vi "Set Btn BG.vi"(8 "error in (no error)":errorcluster, 10 "BG Color":u32(colorbox), 11 "[V] Main UI in":refnum<class "[V] Main UI.lvclass">) -> (0 "error out":errorcluster, 3 "[V] Main UI out":refnum<class "[V] Main UI.lvclass">)   [LabVIEW 2020, in "[V] Main UI.lvlib" / "[V] Main UI.lvclass"]
uses:
  [V] Main UI.lvclass
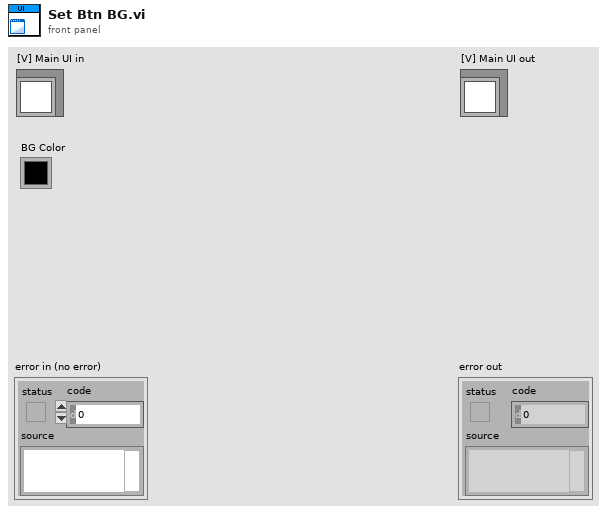
[diagram p1: front panel]
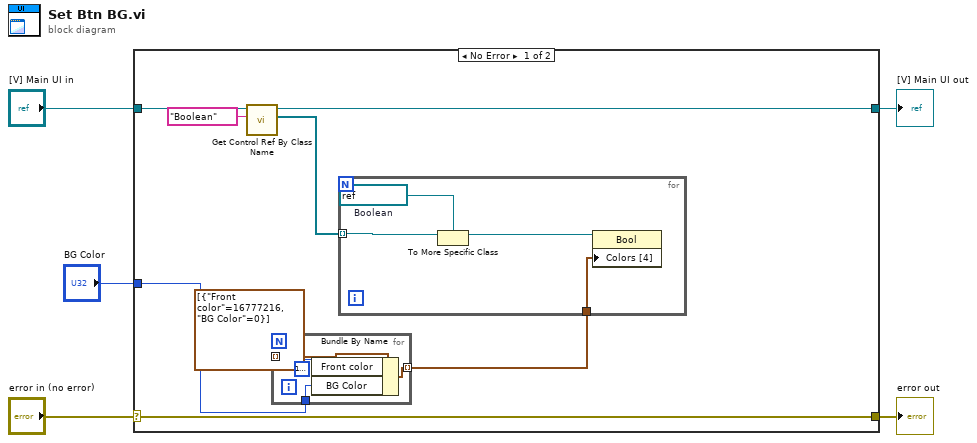
[diagram p0: block diagram]
diagram:
  n1 = case shown="No Error" "error in (no error)" {
    selector: "error in (no error)" -> [w13 w23]
    tunnel: [w13 w23] -> w4
    tunnel: [w10 w22] -> w2
    tunnel: "[V] Main UI in" -> [w12 w22]
    tunnel: "BG Color" -> [w6 _]
    frame No Error {
      n2 = call "Get Control Ref By Class Name.vi"("Control Class"="Boolean", "[V] Main UI in"=w12) -> ("refs"=w9:refnum<vi>[], "[V] Main UI out"=w10:refnum<class "[V] Main UI.lvclass">)  [unwired: 7 in, 1 out]
      n3 = for {
        tunnel: cluster{"Front color":u32, "BG Color":u32}[] [{"Front color"=16777216, "BG Color"=0}] ("Colors [4]") -> [w17] mode=indexing
        tunnel: [w16] -> w7 mode=indexing
        tunnel: w6 -> [w14]
        n4 = Bundle By Name(cluster=w17, "Front color"=u32 16777216, "BG Color"=w14) -> (w16:cluster{"Front color":u32, "BG Color":u32})
      }
      n5 = for {
        tunnel: w9 -> [w21] mode=indexing
        tunnel: w7 -> [w18]
        w20 = refnum<vi> refnum  # Boolean
        n6 = To More Specific Class(target class=w20, reference=w21) -> (specific class reference=w19:refnum<vi>)  [unwired: 1 in, 1 out]
        n7 = property class="Bool"(reference=w19, "Colors [4]"=w18) -> ()  [unwired: 1 in, 2 out]
      }
    }
    frame Error {
    }
  }
  "error out" <- w4
  "[V] Main UI out" <- w2
